vi "Encode Topic Subscriptions.vi"(10 "Topic Subscriptions":T1[](array[typedef])) -> (2 "Payload":u8[](array[numeric]) format="%08b")   [LabVIEW 2013, in "SUBSCRIBE.lvclass"]
uses:
  SUBSCRIBE.lvclass
  Topic Subscription -- cluster.ctl
  ControlPacket/QualityOfService -- enum.ctl
  ControlPacket/ControlPacket.lvclass
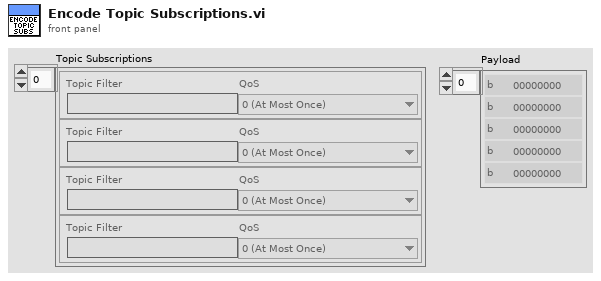
[diagram p1: front panel]
types:
  T1 = typedef "SUBSCRIBE.lvclass/Topic Subscription -- cluster.ctl" = cluster{"Topic Filter":string, "QoS":T2}
  T2 = typedef "ControlPacket.lvclass/QualityOfService -- enum.ctl" = enum16{"0 (At Most Once)", "1 (At Least Once)", "2 (Exactly Once)"}
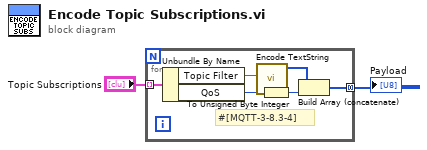
[diagram p0: block diagram]
diagram:
  n1 = for {
    tunnel: "Topic Subscriptions" -> [w8] mode=indexing
    tunnel: [w5] -> w2 mode=concatenating
    # "#[MQTT-3-8.3-4]"
    n2 = Unbundle By Name(w8) -> ("Topic Filter"=w7:string, "QoS"=w4:T2)
    n3 = call "Encode TextString.vi"("Text String"=w7) -> ("Length-Prefixed Field"=w6:u8[])  [unwired: 10 in]
    n4 = To Unsigned Byte Integer(number=w4) -> (unsigned 8bit integer=w3:u8)
    n5 = Build Array (concatenate)(w6, w3) -> (w5:u8[])
  }
  "Payload" <- w2
